vi "Init Board.vi"(8 "error in (no error)":errorcluster, 9 "Columns":u8, 10 "Rows":u8, 11 "Game Engine in":refnum<class "Game Engine.lvclass">) -> (0 "error out":errorcluster, 3 "Game Engine out":refnum<class "Game Engine.lvclass">)   [LabVIEW 2017, in "Game Engine.lvlib" / "Game Engine.lvclass"]
uses:
  Game Engine.lvclass
  Game Engine.lvclass/Game Engine.ctl
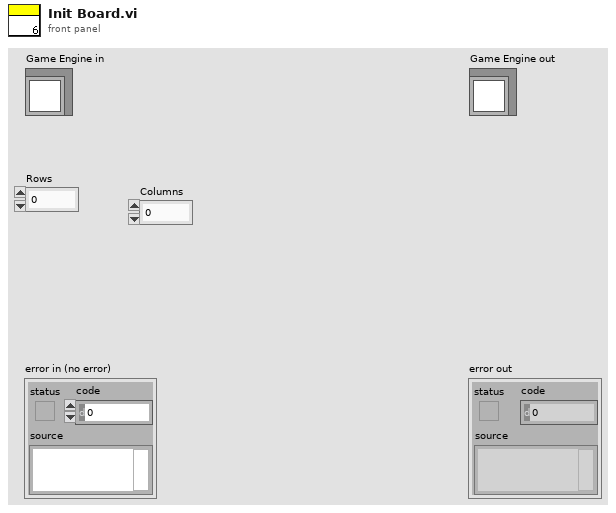
[diagram p1: front panel]
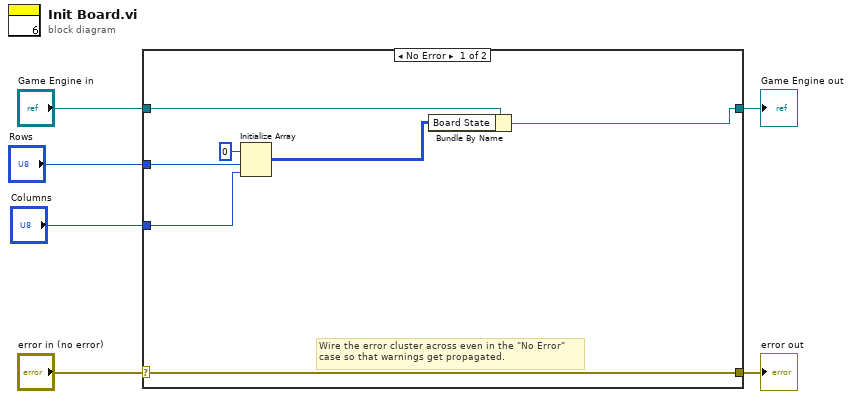
[diagram p0: block diagram]
diagram:
  n1 = case shown="No Error" "error in (no error)" {
    selector: "error in (no error)" -> [w13 w15]
    tunnel: [w13 w15] -> w5
    tunnel: [w7 w14] -> w3
    tunnel: "Game Engine in" -> [w9 w14]
    tunnel: "Rows" -> [w12 _]
    tunnel: "Columns" -> [w11 _]
    frame No Error {
      # "Wire the error cluster across even in the \"No Error\"\ncase so that warnings get propagated."
      n2 = Initialize Array(u32 0 ("element"), w12, w11) -> (w8:u32[][])
      n3 = Bundle By Name(cluster=w9, "Board State"=w8) -> (w7:refnum<class "Game Engine.lvclass">)
    }
    frame Error {
    }
  }
  "error out" <- w5
  "Game Engine out" <- w3
